vi "List Upgradable Packages.vi"(8 "error in":errorcluster) -> (0 "error out":errorcluster, 2 "upgradable packages":string[](array[string]))   [LabVIEW 2014, in "NIPM_API.lvlib"]
doc: "Returns a list of all the versions (from highest to lowest) of the specified package (in all currently registered feeds on this computer)"
uses:
  NIPM_API.lvlib
panel:
  out "cmd standard output":string
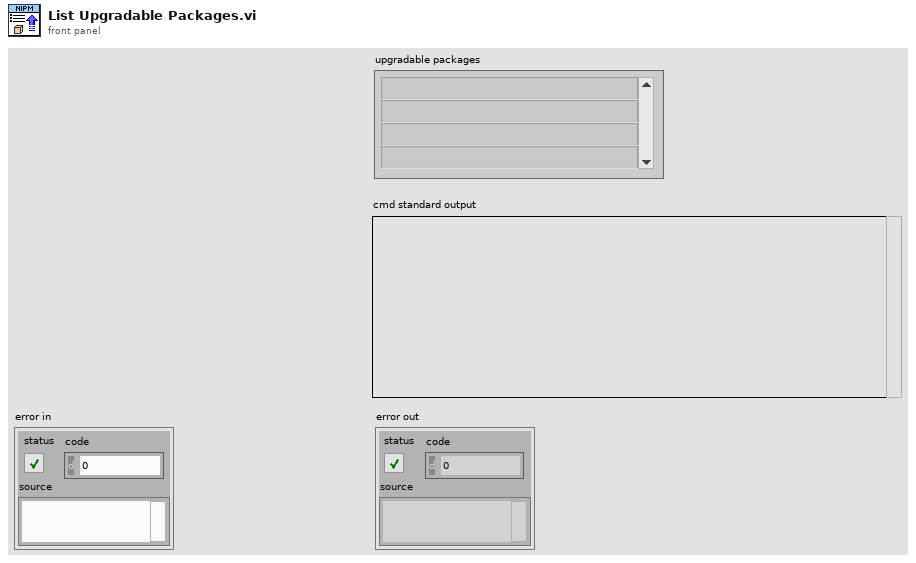
[diagram p1: front panel]
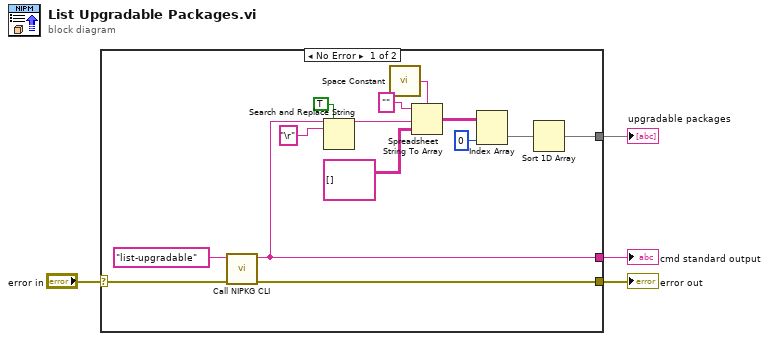
[diagram p0: block diagram]
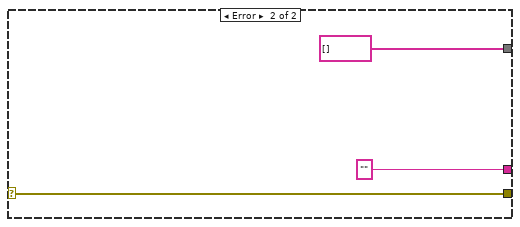
[diagram p2: hidden frame]
diagram:
  n1 = case shown="No Error" "error in" {
    selector: "error in" -> [w7 w21]
    tunnel: [w10 "" ("standard output")] -> w3
    tunnel: [w9 w21] -> w2
    tunnel: [w5 string[] []] -> w1
    frame No Error {
      n2 = call "Call NIPKG CLI.vi"("error in (no error)"=w7, "command"="list-upgradable" ("format string")) -> ("error out"=w9:errorcluster, "command line standard output"=w10:string)  [unwired: 8 in]
      n3 = Search and Replace String(replace all?=TRUE ("replace all? (F)"), input string=w10, search string="\r") -> (result string=w16:string)  [unwired: 5 in, 3 out]
      n4 = call <vilib>:"Space Constant.vi"() -> ("String"=w6:string)
      n5 = Spreadsheet String To Array(delimiter (Tab)=w6, format string="", spreadsheet string=w16, array type (2D Dbl)=string[][] []) -> (array=w13:string[][])
      n6 = Index Array(array=w13, index (col)=0 ("disabled index (col)")) -> (element=w11:string[])  [unwired: 1 in]
      n7 = Sort 1D Array(array=w11) -> (sorted array=w5:string[])
    }
    frame Error {
    }
  }
  "error out" <- w2
  "cmd standard output" <- w3
  "upgradable packages" <- w1
